vi "Apply Ethernet Configuration.vi"(7 "Restart (T)":bool=TRUE, 8 "error in (no error)":errorcluster, 10 "Ethernet Settings":T1={"IP Address"="192.168.1.100", "TCP (Command) Port"=12345, "TCP (Command) Read Interval (ms)"=10, "UDP (Reporting) Port"=54321, "UDP (Reporting) Write Interval (ms)"=5, "UDP Data Broadcast Enable"=FALSE}, 11 "BS120x in":refnum<class "BS120x.lvclass">) -> (0 "error out":errorcluster, 3 "BS120x out":refnum<class "BS120x.lvclass">)   [LabVIEW 2021, in "BS120x Driver.lvlib" / "BS120x.lvclass"]
uses:
  BS120x.lvclass
  TypeDefs/Ethernet Settings.ctl
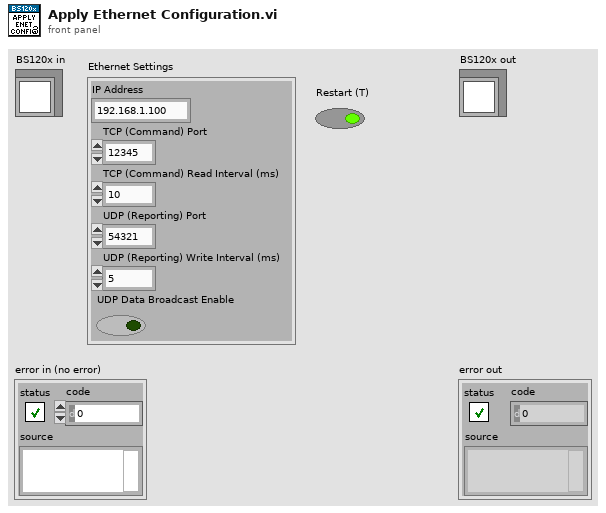
[diagram p1: front panel]
types:
  T1 = typedef "BS120x Driver.lvlib/BS120x.lvclass/Ethernet Settings.ctl" = cluster{"IP Address":string, "TCP (Command) Port":u16, "TCP (Command) Read Interval (ms)":u32, "UDP (Reporting) Port":u16, "UDP (Reporting) Write Interval (ms)":u32, "UDP Data Broadcast Enable":bool}
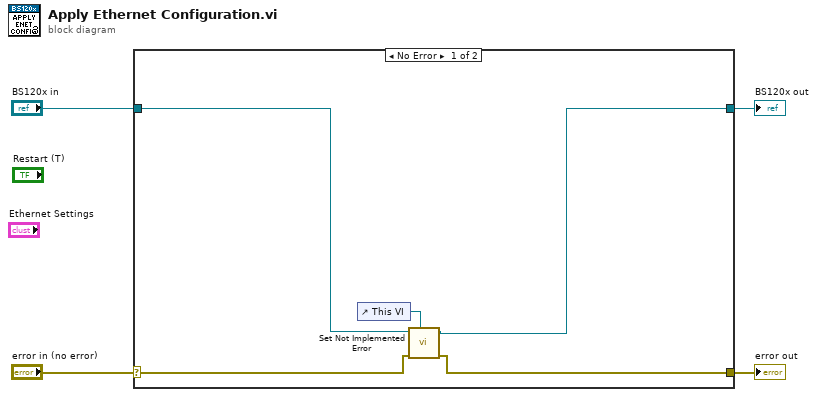
[diagram p0: block diagram]
diagram:
  n1 = case shown="No Error" "error in (no error)" {
    selector: "error in (no error)" -> [w6 w11]
    tunnel: [w5 w11] -> w3
    tunnel: [w7 w10] -> w1
    tunnel: "BS120x in" -> [w8 w10]
    frame No Error {
      n2 = control-ref of="This VI"() -> (w9:refnum<vi>)
      n3 = call "Set Not Implemented Error.vi"("VI Reference"=w9, "error in (no error)"=w6, "BS120x in"=w8) -> ("error out"=w5:errorcluster, "BS120x out"=w7:refnum<class "BS120x.lvclass">)  [unwired: 7 in]
    }
    frame Error {
    }
  }
  "error out" <- w3
  "BS120x out" <- w1
